vi "Read Panel Devices.vi"(8 "error in":errorcluster, 10 "Panel Index":i32, 11 "Manual UI in":refnum<class "Manual UI.lvclass">) -> (0 "error out":errorcluster, 2 "Panel Devices":string[](array[string]), 3 "Manual UI out":refnum<class "Manual UI.lvclass">)   [LabVIEW 2019, in "Manual UI.lvlib" / "Manual UI.lvclass"]
uses:
  Project/Manual UI.lvclass
  Project/Manual UI.lvclass/Manual UI.ctl
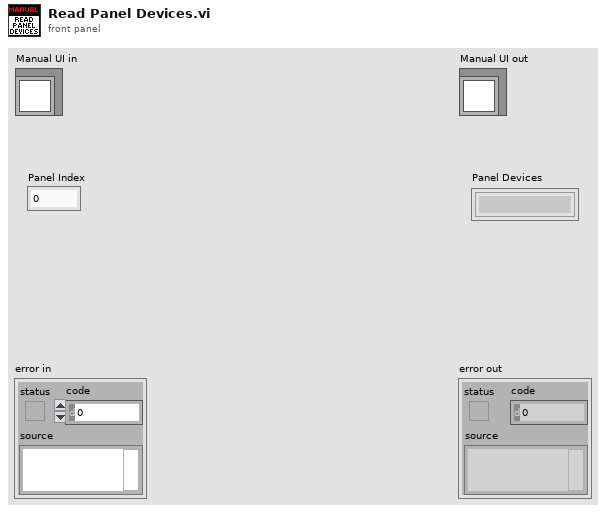
[diagram p1: front panel]
types:
  T1 = cluster{"Name":string, "Instrument":refnum<class "Instruments.lvclass">, "Panel":i32}[]
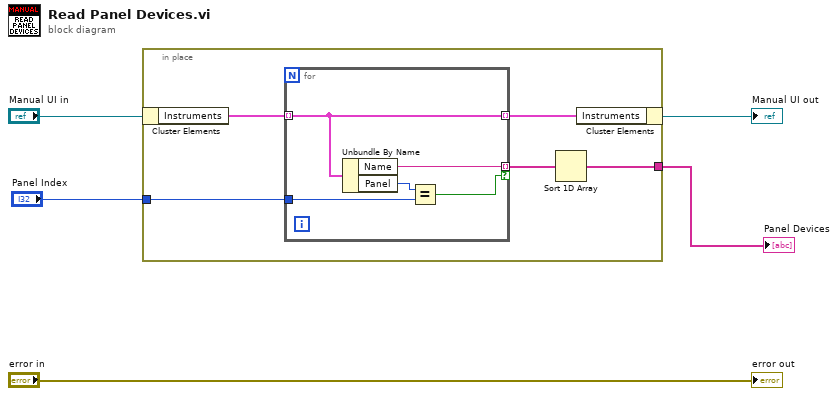
[diagram p0: block diagram]
diagram:
  n1 = in-place {
    in-place-border: "Panel Index" -> [w8]
    in-place-border: [w6] -> w3
    n2 = in-place-cluster #1("Manual UI in") -> ("Instruments"=w10:T1)
    n3 = for {
      tunnel: w10 -> [w15] mode=indexing
      tunnel: [w15] -> w9 mode=indexing
      tunnel: [w14] -> w7 mode=indexing if=w12
      tunnel: w8 -> [w11]
      n4 = Unbundle By Name(w15) -> ("Name"=w14:string, "Panel"=w13:i32)
      n5 = Equal?(x=w13, y=w11) -> (x = y?=w12:bool)
    }
    n6 = Sort 1D Array(array=w7) -> (sorted array=w6:string[])
    n7 = in-place-cluster #1("Instruments"=w9) -> (→"Manual UI out":refnum<class "Manual UI.lvclass">)
  }
  "Panel Devices" <- w3
  "error out" <- "error in"
